vi "comma to tab converter.vi"(2 "System (T: system, F: period)":bool, 7 "',' string":string) -> (8 "'\\t' string":string)   [LabVIEW 2010]
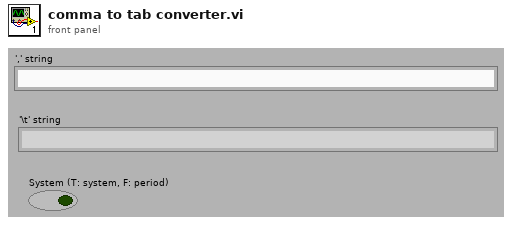
[diagram p1: front panel]
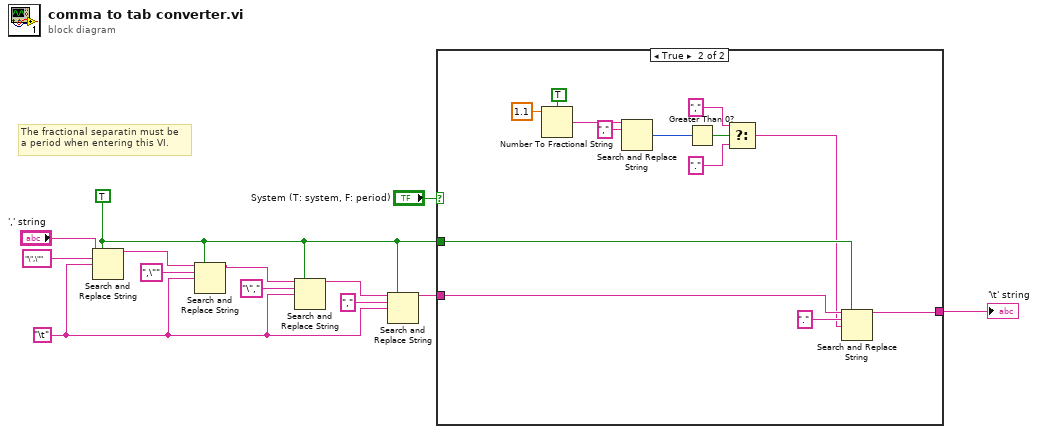
[diagram p0: block diagram]
diagram:
  w3 = TRUE ("replace all? (F)")
  w5 = "\t"
  # "The fractional separatin must be\na period when entering this VI."
  n1 = Search and Replace String(replace all?=w3, input string="',' string", search string="\",\"", replace string=w5) -> (result string=w11:string)  [unwired: 4 in, 3 out]
  n2 = Search and Replace String(replace all?=w3, input string=w11, search string=",\"", replace string=w5) -> (result string=w13:string)  [unwired: 4 in, 3 out]
  n3 = Search and Replace String(replace all?=w3, input string=w13, search string="\",", replace string=w5) -> (result string=w6:string)  [unwired: 4 in, 3 out]
  n4 = Search and Replace String(replace all?=w3, input string=w6, search string=",", replace string=w5) -> (result string=w4:string)  [unwired: 4 in, 3 out]
  n5 = case shown="True" "System (T: system, F: period)" {
    tunnel: w4 -> [w14 w26]
    tunnel: w3 -> [_ w25]
    tunnel: [w14 w15] -> w1
    frame False {
    }
    frame True {
      n6 = Number To Fractional String(use system decimal point (T)=TRUE, number=1.1) -> (F-format string=w22:string)  [unwired: 2 in]
      n7 = Search and Replace String(input string=w22, search string=",") -> (number of replacements=w20:i32)  [unwired: 6 in, 3 out]
      n8 = Greater Than 0?(x=w20) -> (x > 0?=w19:bool)
      n9 = Select(t="," ("search string"), s=w19, f="." ("search string")) -> (s? t:f=w16:string)
      n10 = Search and Replace String(replace all?=w25, input string=w26, search string=".", replace string=w16) -> (result string=w15:string)  [unwired: 4 in, 3 out]
    }
  }
  "'\\t' string" <- w1
